vi "Split Cluster TD.vi"(8 "error in (no error)":errorcluster, 10 "Cluster TD":refnum<class "TD.lvclass">) -> (0 "error out":errorcluster, 2 "element TypeDescriptors":refnum<class "TD.lvclass">[](array[class]))   [LabVIEW 2020, in "variant.lvlib" / "type.lvlib" / "TD.lvclass"]
doc: "Splits the TD of a Cluster into its elements TDs."
uses:
  TD.lvclass
  C:/projects/OpenG-Variant-Data-Library/source/library/Bytes/Bytes.lvclass
  TD.lvclass/TD.ctl
  Bytes/Bytes.lvclass/Bytes.ctl
  Bytes/Bytes.lvclass
  8657b97d-8b19-45af-9c1e-5c12c7aa6ab8.vi
  Bytes/to_data.vi
  get_num_elements.vi/b3898c1b-5169-4cb1-894b-457c92b4a1c3.vi
  8657b97d-8b19-45af-9c1e-5c12c7aa6ab8.vi/81433c74-ee36-47cf-a886-10c868675b30.vi
  8657b97d-8b19-45af-9c1e-5c12c7aa6ab8.vi/d8d9ff34-2c15-4edb-a5ad-7260f11560db.vi
  Bytes/from_byte_array.vi
  get_num_elements.vi/b3898c1b-5169-4cb1-894b-457c92b4a1c3.vi/81433c74-ee36-47cf-a886-10c868675b30.vi
  get_num_elements.vi/b3898c1b-5169-4cb1-894b-457c92b4a1c3.vi/d8d9ff34-2c15-4edb-a5ad-7260f11560db.vi
  Cluster/Cluster.lvclass/Cluster.ctl
  <userlib>/_OpenG.lib/error/error.llb/openg_error.lvlib
  C:/projects/OpenG-Variant-Data-Library/source/library/LVData/Type Descriptor/TD.lvclass
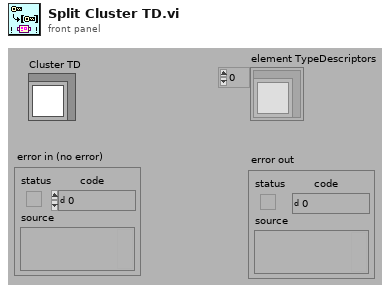
[diagram p1: front panel]
types:
  T1 = typedef "openg_variant.lvlib/Type Descriptor Enumeration.ctl" = enum8{"<Null>", "I8", "I16", "I32", "I64", "U8", "U16", "U32", "U64", "SGL", "DBL", "EXT", "CSG", "CDB", "CXT", "0x0F", "0x10", "0x11", "0x12", "0x13", "0x14", "Enum U8", "Enum U16", "Enum U32", "Enum U64", "SGL PQ", "DBL PQ", "EXT PQ", "CSG PQ", "CDB PQ", "CXT PQ", "0x1F", "0x20", "Boolean", "0x22", "0x23", "0x24", "0x25", "0x26", "0x27", "0x28", "0x29", "0x2A", "0x2B", "0x2C", "0x2D", "0x2E", "0x2F", "String", "0x31", "Path", "Pict", "0x34", "0x35", "0x36", "DAQ", "0x38", "0x39", "0x3A", "0x3B", "0x3C", "0x3D", "0x3E", "0x3F", "Array", "0x41", "0x42", "0x43", "0x44", "0x45", "0x46", "0x47", "0x48", "0x49", "0x4A", "0x4B", "0x4C", "0x4D", "0x4E", "0x4F", "Cluster", "0x51", "0x52", "Variant", "Waveform", "0x55", "0x56", "0x57", "0x58", "0x59", "0x5A", "0x5B", "0x5C", "0x5D", "0x5E", "Fixed Point", "0x60", "0x61", "0x62", "0x63", "0x64", "0x65", "0x66", "0x67", "0x68", "0x69", "0x6A", "0x6B", "0x6C", "0x6D", "0x6E", "0x6F", "Refnum", "0x71", "0x72", "Set Collection", "Map Collection"}
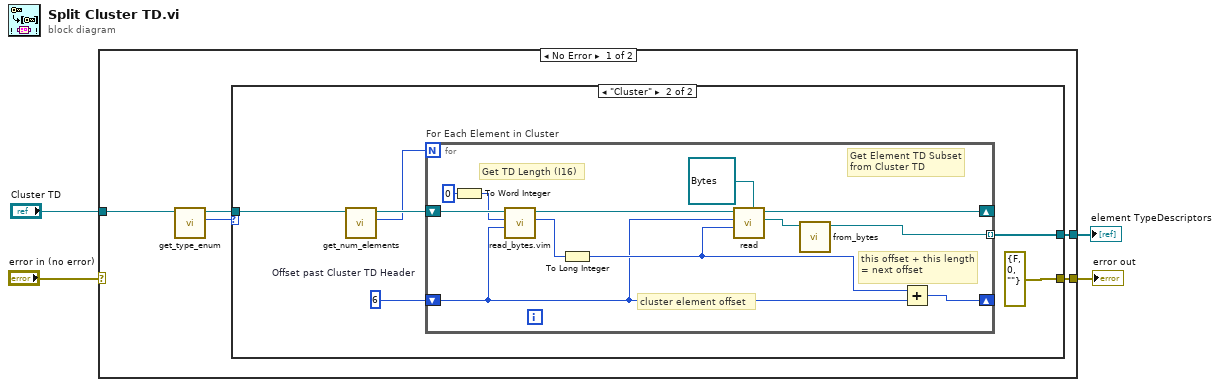
[diagram p0: block diagram]
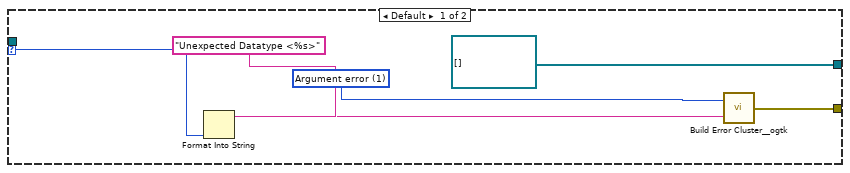
[diagram p2: hidden frame]
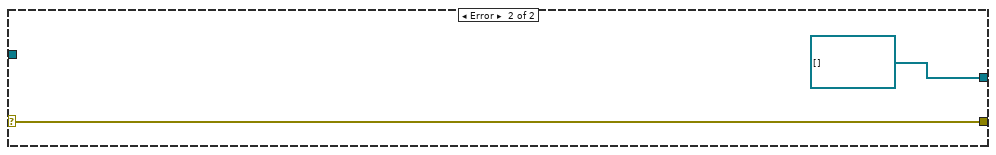
[diagram p3: hidden frame]
diagram:
  n1 = case shown="No Error" "error in (no error)" {
    selector: "error in (no error)" -> [_ w35]
    tunnel: [w9 refnum<class "TD.lvclass">[] []] -> w3
    tunnel: [w8 w35] -> w2
    tunnel: "Cluster TD" -> [w5 _]
    frame No Error {
      n2 = call "get_type_enum.vi"("TypeDescriptor"=w5) -> ("type"=w6:T1, "TypeDescriptor out"=w7:refnum<class "TD.lvclass">)  [unwired: 9 in]
      n3 = case shown="\"Cluster\"" w6 {
        selector: w6 -> [w10 _]
        tunnel: w7 -> [_ w20]
        tunnel: [refnum<class "TD.lvclass">[] [] w19] -> w9
        tunnel: [w14 errorcluster {"status"=FALSE, "code"=0, "source"=""} ("error out")] -> w8
        frame Default {
          w15 = 1 items=["No error", "Argument error", "Memory is full", "Out of zone", "End of file", "File already open", "Generic file I/O error", "File not found", "File permission error", "Disk is full", "Duplicate path", "Too many files open", "System feature not enabled", "Resource file not found", "Cannot add resource", "Resource not found", "Image not found", "Image memory error", "Pen does not exist", "Config type invalid", "Config token not found", "Config parse error", "Config memory error", "Bad external code format", "Bad external code offset", "External code not present", "Null window", "Destroy window error", "Null menu", "Print aborted", "Bad print record", "Print driver error", "Windows error during printing", "Memory error during printing", "Print dialog error", "Generic print error", "Invalid device refnum", "Device not found", "Device parameter error", "Device unit error", "Cannot open device", "Device call aborted", "Generic error", "Cancelled by user", "Object ID too low", "Object ID too high", "Object not in heap", "Unknown heap", "Unknown object (invalid DefProc)", "Unknown object (DefProc not in table)", "Message out of range", "Invalid (null) method", "Unknown message", "Manager call not supported", "Bad address", "Network operation in progress", "Network operation timed out", "Connection is busy", "Network attribute not supported", "Network error", "Address in use", "System out of memory", "Connection aborted", "Connection refused", "Not connected", "Already connected", "Connection closed", "Initialization error (interapplication manager)", "Bad occurrence", "Wait on unbound occurrence handler", "Occurrence queue overflow", "Datalog type conflict", "Unused", "Unrecognized type (interapplication manager)", "Memory corrupt", "Failed to make temporary DLL", "Old CIN version", "Drag socket not found", "Failed to load drop-object", "Failed to register OLE object", "Failed to release OLE object", "Format specifier type mismatch", "Unknown format specifier", "Too few format specifiers", "Too many format specifiers", "Scan failed", "Newer CIN version", "Error converting to variant", "Runtime menu error", "Password tampered", "Variant attribute not found", "Incompatible variant data type", "Event data is not available", "Event Store is not present", "Occurrence is not found", "Event Queue is not created", "Event info is not available", "Refnum passed is NULL", "Error retrieving Class GUID", "Error retrieving CoClass GUID", "Error retrieving TypeLib GUID.", "Bad built application magic bytes.", "Specific driver is different from the specific driver associated with the Logical Name.", "There is no session opened to the class driver.", "Max Error", "MAX - Error with config objects", "MAX - Error loading configuration", "MAX - Group not supported"]
          n4 = Format Into String(format string="Unexpected Datatype <%s>" ("Format String"), w10) -> (resulting string=w11:string)  [unwired: 2 in, 1 out]
          n5 = call <userlib>:"Build Error Cluster__ogtk.vi"("String to Prepend to source (\"\")"=w11, "code"=w15) -> ("error out"=w14:errorcluster)
        }
        frame "Cluster" {
          w21 = 6  # Offset past Cluster TD Header
          n6 = call "get_num_elements.vi"("TypeDescriptor"=w20) -> ("num_element"=w16:i32, "TypeDescriptor out"=w17:refnum<class "TD.lvclass">)  [unwired: 9 in]
          n7 = for "For Each Element in Cluster" {
            N: w16 -> [_]
            shift-right: [w33] -> _
            shift-left: w21 -> [w26]
            tunnel: [w24] -> w19 mode=indexing
            shift-right: [w22] -> _
            shift-left: w17 -> [w32]
            # "Get TD Length (I16)"
            # "this offset + this length = next offset"
            # "cluster element offset"
            # "Get Element TD Subset from Cluster TD"
            n8 = To Word Integer(number=i16 0) -> (16bit integer=w31:i16)
            n9 = call "read_bytes.vim"("byte offset"=w26, "data type"=w31, "Bytes in"=w32) -> ("value"=w29:i16, "Bytes out"=w28:refnum<class "TD.lvclass">)  [unwired: 7 in]
            n10 = To Long Integer(number=w29) -> (32bit integer=w27:i32)
            n11 = call "read.vi"("type to read"=refnum<class "Bytes.lvclass"> refnum, "length (-1: rest)"=w27, "offset (-1: current position)"=w26, "Bytes in"=w28) -> ("Bytes read"=w23:refnum<class "Bytes.lvclass">, "Bytes out"=w22:refnum<class "TD.lvclass">)  [unwired: 6 in]
            n12 = call "from_bytes.vi"("Bytes"=w23) -> ("TypeDescriptor"=w24:refnum<class "TD.lvclass">)  [unwired: 10 in]
            n13 = Add(x=w27, y=w26) -> (x+y=w33:i32)
          }
        }
      }
    }
    frame Error {
    }
  }
  "error out" <- w2
  "element TypeDescriptors" <- w3
